vi "Configure CALC2 Math Calculation.vi"(8 "error in (no error)":errorcluster, 9 "Enable CALC 2 Calculation (T: Enable)":bool=TRUE, 10 "Calculation Format (5: NONE)":i32(ring)=5 items=["Mean", "Standard Deviation", "MAX", "MIN", "Peak-to-peak", "NONE"], 11 "VISA resource name":refnum<visa-resource-name>) -> (0 "error out":errorcluster, 3 "VISA resource name out":refnum<visa-resource-name>)   [LabVIEW 2020, in "Keithley 6517.lvlib"]
doc: "Enables or disables the CALC 2 calculation and configures the format for the CALC 2 math calculation.\n\n<B>Note:</B>\nThis VI is <B>NOT</B> compatible with model <B>6514</B>."
uses:
  <instrlib>/Keithley 6517/Keithley 6517.lvlib
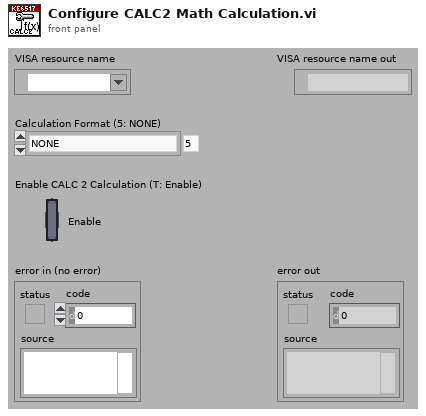
[diagram p1: front panel]
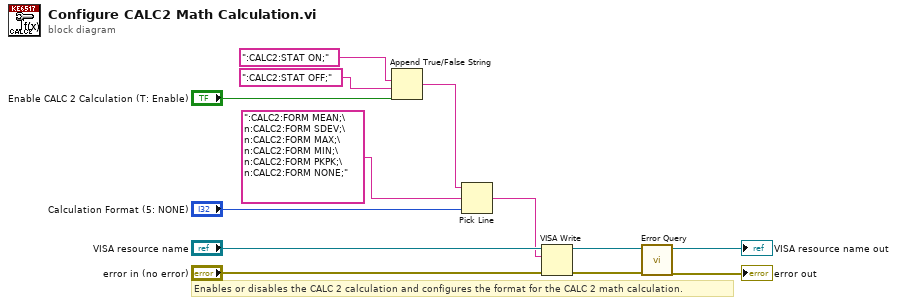
[diagram p0: block diagram]
diagram:
  # "Enables or disables the CALC 2 calculation and configures the format for the CALC 2 math calculation."
  n1 = Append True/False String(1:"Enable CALC 2 Calculation (T: Enable)", 2:":CALC2:STAT OFF;", 3:":CALC2:STAT ON;") -> (0:w2:string)  [unwired: 1 in]
  n2 = Pick Line(string ("")=w2, multi-line string=":CALC2:FORM MEAN;\n:CALC2:FORM SDEV;\n:CALC2:FORM MAX;\n:CALC2:FORM MIN;\n:CALC2:FORM PKPK;\n:CALC2:FORM NONE;", line index="Calculation Format (5: NONE)") -> (output string=w1:string)
  n3 = VISA Write(VISA resource name="VISA resource name", write buffer=w1, error in (no error)="error in (no error)") -> (VISA resource name out=w8:refnum<visa-resource-name>, error out=w7:errorcluster)  [unwired: 1 out]
  n4 = call <instrlib>:"Error Query.vi"("error in (no error)"=w7, "VISA resource name"=w8) -> ("error out"=→"error out":errorcluster, "VISA resource name out"=→"VISA resource name out":refnum<visa-resource-name>)  [unwired: 6 in, 2 out]
